vi "Test.labview.mqtt.vi"() -> ()   [LabVIEW 2014]
uses:
  mqtt/mqttTypedef/mqttConnectionStatus.ctl
  mqtt/mqttTypedef/mqttBroker.ctl
  mqtt/mqttTypedef/mqttConnectionFlags.ctl
  mqtt/mqttTypedef/mqttWillInformation.ctl
  mqtt/mqttTypedef/mqttSubscribeCluster.ctl
  mqtt/mqttTypedef/mqttQOSlevel.ctl
  mqtt/mqtt.lvclass
  labview-mqtt.lvlib
panel:
  out "HISTORY":string
  in  "STATUS/XYZMN":dbl[](array[numeric])=[0.0, 0.0, 0.0, 0.0, 0.0]
  in  "STATUS/abcdefg":dbl[](array[numeric])=[0.0, 0.0, 0.0, 0.0, 0.0]
  in  "STATUS/FollowEnable":bool
  in  "STATUS/Up_Enable":bool
  out "success":bool
  out "sessionPresent":bool
  out "connStatus":T1
  out "Error":errorcluster
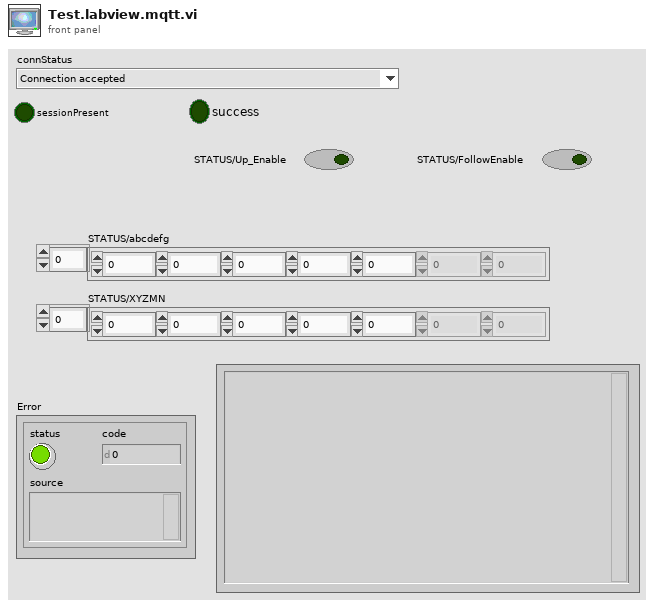
[diagram p1: front panel]
types:
  T1 = typedef "labview-mqtt.lvlib/mqttConnectionStatus.ctl" = enum16{"Connection accepted", "Connection refused: unacceptable protocol version", "Connection refused: identifier rejected", "Connection refused: Server unavailable", "Connection refused: bad user name or password", "Connection refused: not authorized"}
  T2 = typedef "labview-mqtt.lvlib/mqttSubscribeCluster.ctl" = cluster{"Topic":string, "QoS":T3}
  T3 = typedef "labview-mqtt.lvlib/mqttQOSlevel.ctl" = enum8{"At most once", "At least once", "Exactly once", "Reserved"}
  T4 = typedef "labview-mqtt.lvlib/mqttWillInformation.ctl" = cluster{"User Name":string, "Password":string}
  T5 = typedef "labview-mqtt.lvlib/mqttConnectionFlags.ctl" = cluster{"reserved":bool, "clean session":bool, "will flag":bool, "willQOS":enum8{"At most once", "At least once", "Exactly once", "Reserved"}, "will retain":bool, "password":bool, "user name":bool}
  T6 = typedef "labview-mqtt.lvlib/mqttBroker.ctl" = cluster{"address":string, "port":u16, "connTimeout":i32, "writeTimeout":i32, "readTimeout":i32, "subTimeout":i32}
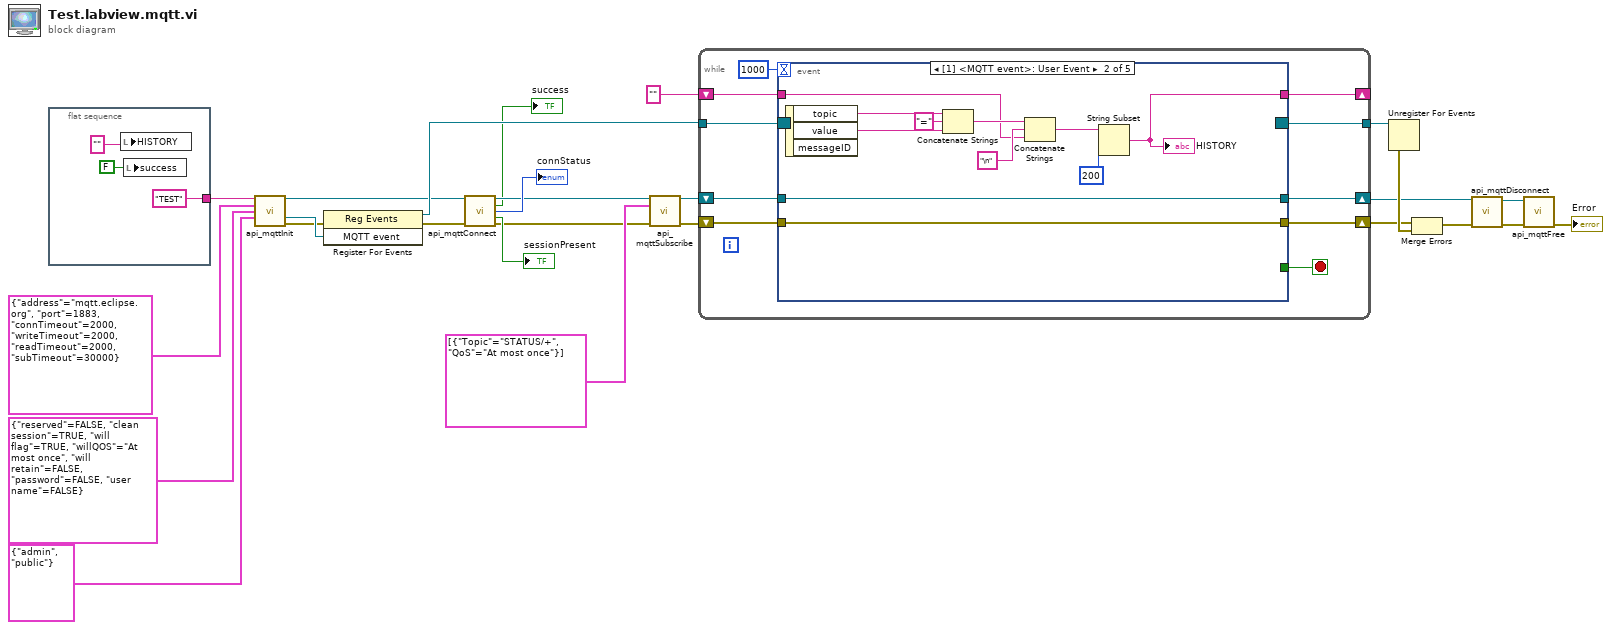
[diagram p0: block diagram]
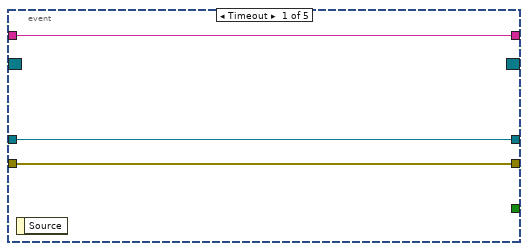
[diagram p2: hidden frame]
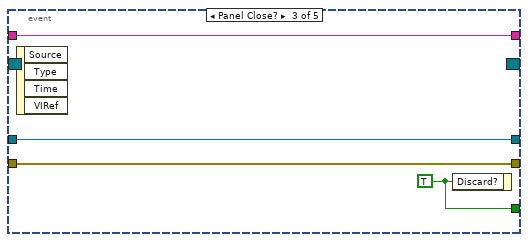
[diagram p3: hidden frame]
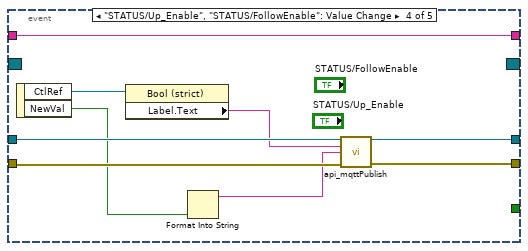
[diagram p4: hidden frame]
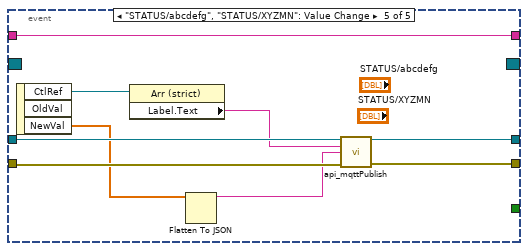
[diagram p5: hidden frame]
diagram:
  n1 = flat-sequence {
    tunnel: ["TEST" ("client")] -> w4
    frame #0 {
      n2 = local write "HISTORY"("" ("HISTORY")) -> ()
      n3 = local write "success"(FALSE ("success")) -> ()
    }
  }
  n4 = call "api_mqttInit.vi"("client"=w4, "broker"=T6 {"address"="mqtt.eclipse.org", "port"=1883, "connTimeout"=2000, "writeTimeout"=2000, "readTimeout"=2000, "subTimeout"=30000}, "connFlags"=T5 {"reserved"=FALSE, "clean session"=TRUE, "will flag"=TRUE, "willQOS"=enum."At most once", "will retain"=FALSE, "password"=FALSE, "user name"=FALSE}, "User Info"=T4 {"User Name"="admin", "Password"="public"}) -> ("mqtt.lvclass out"=w6:refnum<class "mqtt.lvclass">, "MQTT event"=w20:refnum<user-event>, "error out"=w19:errorcluster)  [unwired: 9 in]
  n5 = register-events(error in=w19, w20) -> (reference out=w26:refnum<event-registration>, error out=w5:errorcluster)  [unwired: 1 in]
  n6 = call "api_mqttConnect.vi"("mqtt.lvclass in"=w6, "error in (no error)"=w5) -> ("mqtt.lvclass out"=w15:refnum<class "mqtt.lvclass">, "success"=→"success":bool, "connStatus"=→"connStatus":T1, "sessionPresent"=→"sessionPresent":bool, "error out"=w14:errorcluster)  [unwired: 9 in]
  n7 = call "api_mqttSubscribe.vi"("mqtt.lvclass in"=w15, "subscriptionInfo"=T2[] [{"Topic"="STATUS/+", "QoS"=enum."At most once"}], "error in (no error)"=w14) -> ("mqtt.lvclass out"=w7:refnum<class "mqtt.lvclass">, "error out"=w13:errorcluster)  [unwired: 10 in, 1 out]
  n8 = while {
    shift-right: [w38] -> w10
    shift-left: w7 -> [w39]
    shift-right: [w33] -> w23
    shift-left: w13 -> [w37]
    tunnel: w26 -> [w36]
    tunnel: [w35] -> w25
    shift-right: [w31] -> _
    shift-left: "" ("string") -> [w32]
    stop <- w30 stop-if-true
    n9 = event shown="[1] <MQTT event>: User Event" {
      selector: w36 -> [_ _ _ _ _]
      dyn-events: [_ _ _ _ _] -> w35
      timeout: 1000 -> [_ _ _ _ _]
      tunnel: w39 -> [w42 w53 w57 w66 w75]
      tunnel: [w42 w53 w57 w64 w73] -> w38
      tunnel: w37 -> [w41 w52 w56 w65 w74]
      tunnel: [w41 w52 w56 w63 w72] -> w33
      tunnel: w32 -> [w40 w45 w55 w58 w67]
      tunnel: [w40 w43 w55 w58 w67] -> w31
      tunnel: [_ _ w54 _ _] -> w30
      event Timeout {
        n10 = event-data() -> ()  [unwired: 1 in, 1 out]
      }
      event User Event {
        n11 = event-data() -> ("topic"=w51:string, "value"=w50:string)  [unwired: 1 in, 1 out]
        n12 = Concatenate Strings(w51, "=" ("string"), w50) -> (w46:string)
        n13 = Concatenate Strings(w46, "\n" ("string"), w45) -> (w47:string)
        n14 = String Subset(string=w47, length (rest)=200 ("length (rest)")) -> (substring=w43:string)  [unwired: 1 in]
        "HISTORY" <- w43
      }
      event Panel Close? {
        w54 = TRUE ("Discard?")
        n15 = event-data() -> ()  [unwired: 1 in, 4 out]
        n16 = event-data("Discard?"=w54) -> ()  [unwired: 1 in, 1 out]
      }
      event "STATUS/Up_Enable", "STATUS/FollowEnable": Value Change {
        n17 = event-data() -> ("CtlRef"=w62:refnum<vi>, "NewVal"=w60:bool)  [unwired: 1 in]
        n18 = property class="Bool (strict)"(reference=w62) -> ("Label.Text"=w61:string)  [unwired: 1 in, 2 out]
        n19 = Format Into String(w60) -> (resulting string=w59:string)  [unwired: 3 in, 1 out]
        n20 = call "api_mqttPublish.vi"("mqtt.lvclass in"=w66, "topic"=w61, "value"=w59, "error in (no error)"=w65) -> ("mqtt.lvclass out"=w64:refnum<class "mqtt.lvclass">, "error out"=w63:errorcluster)  [unwired: 9 in, 1 out]
      }
      event "STATUS/abcdefg", "STATUS/XYZMN": Value Change {
        n21 = event-data() -> ("CtlRef"=w71:refnum<vi>, "NewVal"=w69:dbl[])  [unwired: 1 in, 1 out]
        n22 = property class="Arr (strict)"(reference=w71) -> ("Label.Text"=w70:string)  [unwired: 1 in, 2 out]
        n23 = Flatten To JSON(anything=w69) -> (JSON string=w68:string)  [unwired: 2 in, 1 out]
        n24 = call "api_mqttPublish.vi"("mqtt.lvclass in"=w75, "topic"=w70, "value"=w68, "error in (no error)"=w74) -> ("mqtt.lvclass out"=w73:refnum<class "mqtt.lvclass">, "error out"=w72:errorcluster)  [unwired: 9 in, 1 out]
      }
    }
  }
  n25 = Unregister For Events(event registration refnum=w25) -> (error out=w24:errorcluster)  [unwired: 1 in]
  n26 = Merge Errors(w23, w24) -> (w9:errorcluster)
  n27 = call "api_mqttDisconnect.vi"("mqtt.lvclass in"=w10, "error in (no error)"=w9) -> ("mqtt.lvclass out"=w12:refnum<class "mqtt.lvclass">, "error out"=w11:errorcluster)  [unwired: 11 in, 1 out]
  n28 = call "api_mqttFree.vi"("error in (no error)"=w11, "mqtt in"=w12) -> ("error out"=→"Error":errorcluster)  [unwired: 8 in, 1 out]
